vi "Semi Auto Intake Mode.vi"(9 "Current Intake Angle":dbl) -> (1 "Intake Open":bool, 2 "Intake Right Power":dbl, 3 "Intake Left Power":dbl, 4 "Intake Angle":dbl, 5 "Intake States":T1)   [LabVIEW 2017]
uses:
  Common Code/Intake States.ctl
  Robot Global Data.vi
  <vilib>/addons/control/pid/pid.llb/PID (DBL).vi
  <vilib>/addons/control/pid/NI_PID_pid.lvlib
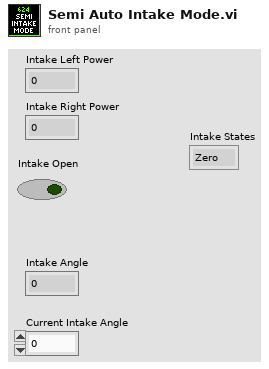
[diagram p1: front panel]
types:
  T1 = typedef "Intake States.ctl" = enum16{"Zero", "Override Angle", "Idle", "Drop Mid", "Drop Low", "Outtake", "Intake"}
  T2 = typedef "Drivetrain Settings Cluster.ctl" = cluster{"Gyro Steer PID Gains":T3, "Distance Drive PID Gains":T3, "Drive Tolerance":dbl, "Gyro Tolerance":dbl, "Gyro Output":dbl, "Distance Output":dbl, "Y Power Multiplier":dbl, "Turn Power Multiplier":dbl, "Creep Rate":dbl, "Constant Power":bool, "DT Mode Modifier":enum16{"None, Default", "Cube", "Square"}, "Left Encoder Tick Constant":dbl, "Right Encoder Tick Constant":dbl, "Shift Speed":dbl}
  T3 = typedef "PID Gains Cluster.ctl" = cluster{"Integral Time":dbl, "Proportional Gain":dbl, "Derivative Time":dbl}
  T4 = typedef "Intake Presets.ctl" = cluster{"Idle Angle":dbl, "Mid Angle":dbl, "Low Angle":dbl, "Outtake Power":dbl, "Intake Power":dbl, "Unstuck":dbl, "Angle Tolerance":dbl, "Max Angle":dbl, "Max Current":dbl, "Current Trip Time":dbl, "Reset Encoder?":bool, "Encoder Scale":dbl, "PID gains":cluster{"proportional gain (Kc)":dbl, "integral time (Ti, min)":dbl, "derivative time (Td, min)":dbl}, "output range":cluster{"output high":dbl, "output low":dbl}}
  T5 = typedef "Elevator Settings Cluster.ctl" = cluster{"Ground Height":dbl, "Switch Height":dbl, "Scale High Height ":dbl, "Scale Low Height":dbl, "Elevator PID Gains":T6, "Elevator Tolerance":dbl, "Reset Encoders":bool, "Encoder Scale":dbl, "Max Height":dbl, "Mid Height":dbl, "output range":cluster{"output high":dbl, "output low":dbl}}
  T6 = typedef "PID Gains.ctl" = cluster{"proportional gain (Kc)":dbl, "integral time (Ti, min)":dbl, "derivative time (Td, min)":dbl}
  T7 = cluster{"Drivetrain Settings Cluster":T2, "Intake Presets":T4, "Elevator Settings Cluster":T5}
  T8 = typedef "Elevator Status Cluster.ctl" = cluster{"Finished":bool, "Output":dbl, "Elevator State":T9, "Elevator Mode":T10, "Encoder Height":dbl, "Elevator Height":dbl, "At Bottom?":bool, "At Top?":bool}
  T9 = typedef "Elevator State.ctl" = enum16{"Idle", "Ground", "Mid", "Scale", "Switch"}
  T10 = typedef "Elevator Mode.ctl" = enum16{"Semi Auto", "Manual", "Auto"}
  T11 = typedef "Intake Command Cluster.ctl" = cluster{"Intake Mode":T12, "Intake States":T1, "Manual Roller Power":dbl, "Manual Close?":bool, "Manual Lift Power":dbl, "Override Lift?":bool, "Override Angle":dbl}
  T12 = typedef "Intake Mode.ctl" = enum16{"Auto", "Semi Auto", "Manual"}
  T13 = cluster{"proportional gain (Kc)":dbl, "integral time (Ti, min)":dbl, "derivative time (Td, min)":dbl}
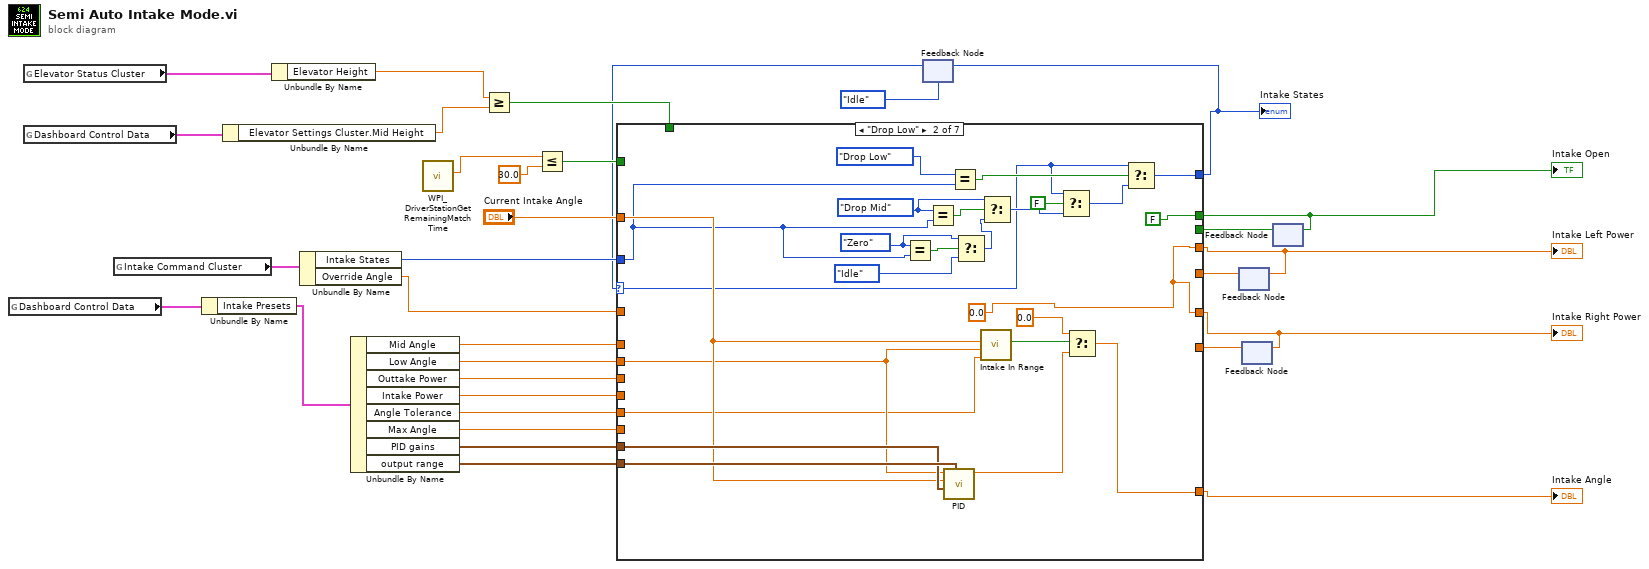
[diagram p0: block diagram]
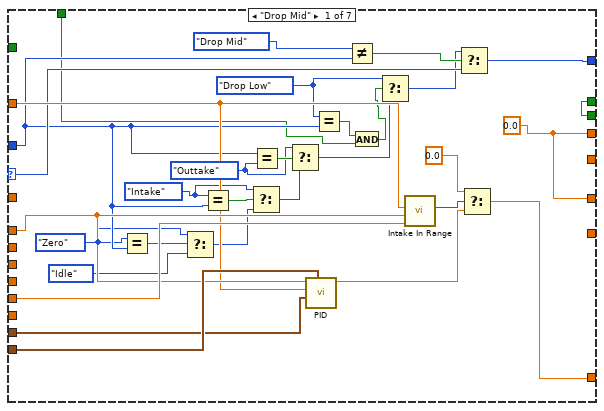
[diagram p2: hidden frame]
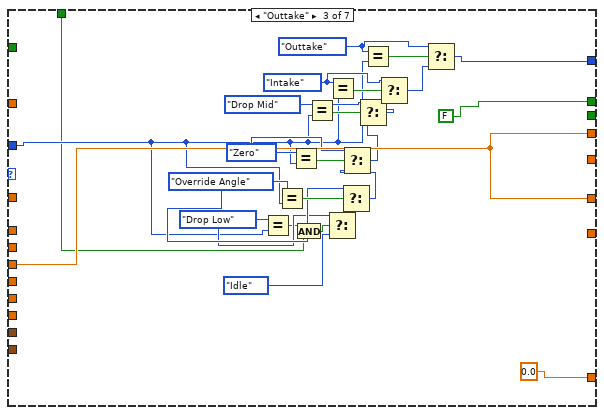
[diagram p3: hidden frame]
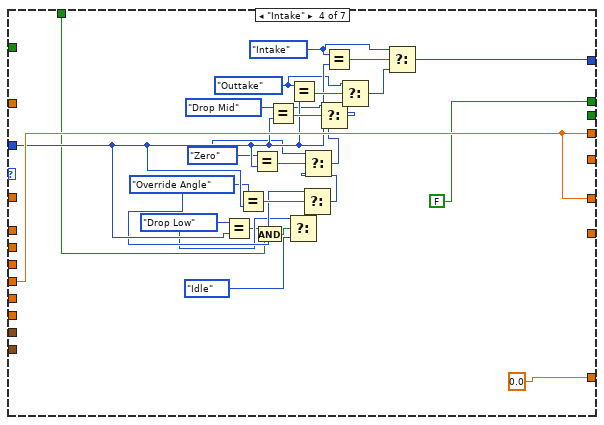
[diagram p4: hidden frame]
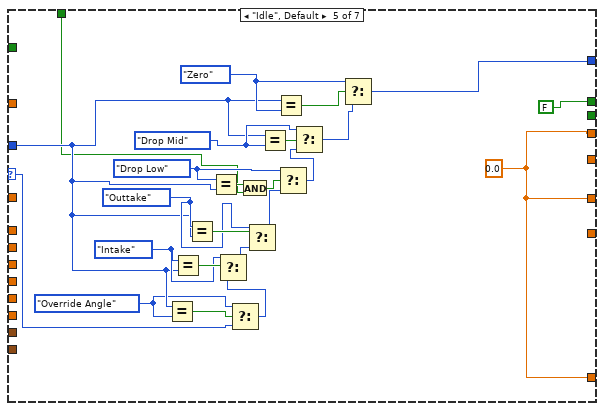
[diagram p5: hidden frame]
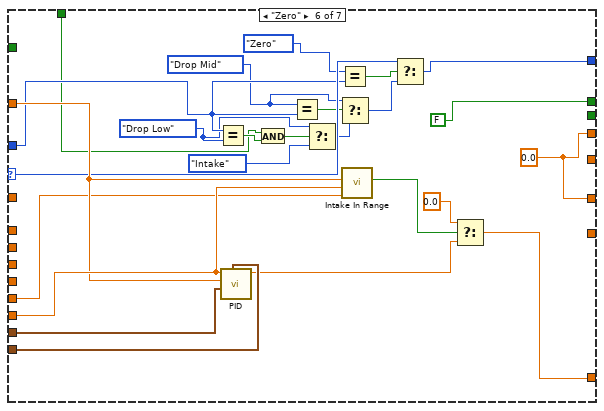
[diagram p6: hidden frame]
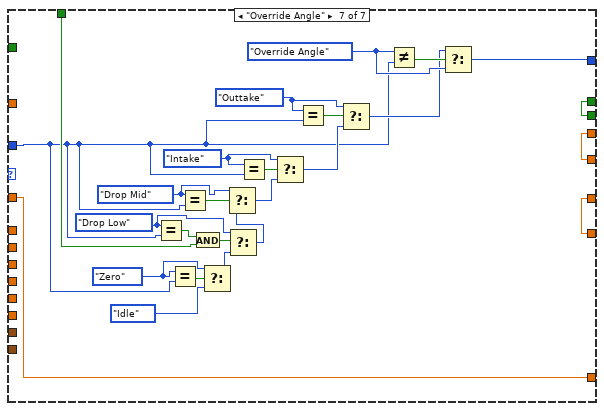
[diagram p7: hidden frame]
diagram:
  n1 = global read "Robot Global Data.vi" "Dashboard Control Data"() -> (w30:T7)
  n2 = global read "Robot Global Data.vi" "Elevator Status Cluster"() -> (w18:T8)
  n3 = global read "Robot Global Data.vi" "Dashboard Control Data"() -> (w17:T7)
  n4 = global read "Robot Global Data.vi" "Intake Command Cluster"() -> (w32:T11)
  n5 = Unbundle By Name(w30) -> ("Intake Presets"=w29:T4)
  n6 = Unbundle By Name(w17) -> ("Elevator Settings Cluster.Mid Height"=w15:dbl)
  n7 = Unbundle By Name(w18) -> ("Elevator Height"=w16:dbl)
  n8 = Unbundle By Name(w32) -> ("Intake States"=w31:T1, "Override Angle"=w7:dbl)
  n9 = Unbundle By Name(w29) -> ("Mid Angle"=w28:dbl, "Low Angle"=w27:dbl, "Outtake Power"=w26:dbl, "Intake Power"=w25:dbl, "Angle Tolerance"=w24:dbl, "Max Angle"=w23:dbl, "PID gains"=w22:T13, "output range"=w21:cluster{"output high":dbl, "output low":dbl})
  n10 = call <vilib>:"WPI_DriverStationGetRemainingMatchTime.vi"() -> ("Match Time(s)"=w13:sgl)  [unwired: 10 in, 1 out]
  n11 = Greater Or Equal?(x=w16, y=w15) -> (x >= y?=w14:bool)
  n12 = Less Or Equal?(x=w13, y=30.0) -> (x <= y?=w11:bool)
  n13 = feedback #1(Intake_States."Idle" ("Intake States")) -> (w8:T1)
  n14 = feedback #2() -> (w5:dbl)  [unwired: 1 in]
  n15 = feedback #3() -> (w3:dbl)  [unwired: 1 in]
  n16 = feedback #4() -> (w9:bool)  [unwired: 1 in]
  n17 = case shown="\"Drop Low\"" w8 {
    selector: w8 -> [w51 w73 _ _ w141 w175 _]
    tunnel: w31 -> [w41 w67 w91 w129 w147 w173 w193]
    tunnel: [w37 w71 w90 w114 w152 w164 w188] -> w1
    tunnel: [w33 FALSE FALSE FALSE FALSE FALSE w212] -> w10
    tunnel: [w54 w66 w112 w138 w148 w178 w211] -> w6
    tunnel: [w54 w66 w112 w138 w148 w178 w210] -> w4
    tunnel: [w55 w83 0.0 0.0 w148 w179 w213] -> w19
    tunnel: w28 -> [w60 _ _ _ _ _ _]
    tunnel: w27 -> [_ w81 _ _ _ _ _]
    tunnel: w26 -> [_ _ w112 _ _ _ _]
    tunnel: w25 -> [_ _ _ w138 _ _ _]
    tunnel: w24 -> [w61 w80 _ _ _ w183 _]
    tunnel: w23 -> [_ _ _ _ _ w185 _]
    tunnel: w22 -> [w62 w87 _ _ _ w187 _]
    tunnel: w21 -> [w63 w88 _ _ _ w186 _]
    tunnel: "Current Intake Angle" -> [w59 w82 _ _ _ w184 _]
    tunnel: w14 -> [w34 _ w89 w117 w145 w171 w198]
    tunnel: w11 -> [_ _ _ _ _ _ _]
    tunnel: w9 -> [w33 _ _ _ _ _ w212]
    tunnel: w7 -> [_ _ _ _ _ _ w213]
    tunnel: w5 -> [_ _ _ _ _ _ w211]
    tunnel: w3 -> [_ _ _ _ _ _ w210]
    frame "Drop Mid" {
      w40 = Intake_States."Zero" ("Intake States")
      w44 = Intake_States."Intake" ("Intake States")
      w48 = Intake_States."Outtake" ("Intake States")
      w50 = Intake_States."Drop Low" ("Intake States")
      w54 = 0.0
      n18 = Equal?(x=w40, y=w41) -> (x = y?=w42:bool)
      n19 = Select(t=w40, s=w42, f=Intake_States."Idle" ("Intake States")) -> (s? t:f=w38:T1)
      n20 = Equal?(x=w44, y=w41) -> (x = y?=w45:bool)
      n21 = Select(t=w44, s=w45, f=w38) -> (s? t:f=w43:T1)
      n22 = Equal?(x=w41, y=w48) -> (x = y?=w49:bool)
      n23 = Select(t=w48, s=w49, f=w43) -> (s? t:f=w47:T1)
      n24 = call-poly <vilib>:"PID.vi"("output range"=w63, "PID gains"=w62, "process variable"=w59, "setpoint"=w60) -> ("output"=w57:dbl)  [unwired: 6 in, 1 out]
      n25 = Equal?(x=w50, y=w41) -> (x = y?=w36:bool)
      n26 = Not Equal?(x=Intake_States."Drop Mid" ("Intake States"), y=w41) -> (x != y?=w52:bool)
      n27 = And(x=w36, y=w34) -> (x .and. y?=w35:bool)
      n28 = Select(t=w50, s=w35, f=w47) -> (s? t:f=w46:T1)
      n29 = call "Intake In Range.vi"("Angle Tolerance"=w61, "Target Height"=w60, "Actual Height"=w59) -> ("In Range?"=w58:bool)  [unwired: 8 in]
      n30 = Select(t=w46, s=w52, f=w51) -> (s? t:f=w37:T1)
      n31 = Select(t=0.0, s=w58, f=w57) -> (s? t:f=w55:dbl)
    }
    frame "Drop Low" {
      w66 = 0.0
      w70 = Intake_States."Zero" ("Intake States")
      w76 = Intake_States."Drop Mid" ("Intake States")
      n32 = Equal?(x=w70, y=w67) -> (x = y?=w75:bool)
      n33 = Equal?(x=w76, y=w67) -> (x = y?=w77:bool)
      n34 = call-poly <vilib>:"PID.vi"("output range"=w88, "PID gains"=w87, "process variable"=w82, "setpoint"=w81) -> ("output"=w85:dbl)  [unwired: 6 in, 1 out]
      n35 = Equal?(x=Intake_States."Drop Low" ("Intake States"), y=w67) -> (x = y?=w78:bool)
      n36 = Select(t=w70, s=w75, f=Intake_States."Idle" ("Intake States")) -> (s? t:f=w69:T1)
      n37 = call "Intake In Range.vi"("Angle Tolerance"=w80, "Target Height"=w81, "Actual Height"=w82) -> ("In Range?"=w86:bool)  [unwired: 8 in]
      n38 = Select(t=w76, s=w77, f=w69) -> (s? t:f=w74:T1)
      n39 = Select(t=w73, s=FALSE, f=w74) -> (s? t:f=w72:T1)
      n40 = Select(t=0.0, s=w86, f=w85) -> (s? t:f=w83:dbl)
      n41 = Select(t=w73, s=w78, f=w72) -> (s? t:f=w71:T1)
    }
    frame "Outtake" {
      w100 = Intake_States."Drop Low" ("Intake States")
      w101 = Intake_States."Override Angle" ("Intake States")
      w102 = Intake_States."Zero" ("Intake States")
      w103 = Intake_States."Drop Mid" ("Intake States")
      w104 = Intake_States."Intake" ("Intake States")
      w109 = Intake_States."Outtake" ("Intake States")
      n42 = Equal?(x=w100, y=w91) -> (x = y?=w94:bool)
      n43 = Equal?(x=w101, y=w91) -> (x = y?=w105:bool)
      n44 = Equal?(x=w102, y=w91) -> (x = y?=w106:bool)
      n45 = And(x=w94, y=w89) -> (x .and. y?=w93:bool)
      n46 = Equal?(x=w103, y=w91) -> (x = y?=w107:bool)
      n47 = Select(t=w100, s=w93, f=Intake_States."Idle" ("Intake States")) -> (s? t:f=w95:T1)
      n48 = Equal?(x=w104, y=w91) -> (x = y?=w108:bool)
      n49 = Select(t=w101, s=w105, f=w95) -> (s? t:f=w96:T1)
      n50 = Select(t=w102, s=w106, f=w96) -> (s? t:f=w97:T1)
      n51 = Select(t=w103, s=w107, f=w97) -> (s? t:f=w99:T1)
      n52 = Equal?(x=w109, y=w91) -> (x = y?=w110:bool)
      n53 = Select(t=w104, s=w108, f=w99) -> (s? t:f=w98:T1)
      n54 = Select(t=w109, s=w110, f=w98) -> (s? t:f=w90:T1)
    }
    frame "Intake" {
      w124 = Intake_States."Drop Low" ("Intake States")
      w125 = Intake_States."Override Angle" ("Intake States")
      w126 = Intake_States."Zero" ("Intake States")
      w127 = Intake_States."Drop Mid" ("Intake States")
      w128 = Intake_States."Outtake" ("Intake States")
      w134 = Intake_States."Intake" ("Intake States")
      n55 = Equal?(x=w124, y=w129) -> (x = y?=w118:bool)
      n56 = Equal?(x=w125, y=w129) -> (x = y?=w130:bool)
      n57 = Equal?(x=w126, y=w129) -> (x = y?=w131:bool)
      n58 = And(x=w118, y=w117) -> (x .and. y?=w116:bool)
      n59 = Equal?(x=w127, y=w129) -> (x = y?=w132:bool)
      n60 = Select(t=w124, s=w116, f=Intake_States."Idle" ("Intake States")) -> (s? t:f=w119:T1)
      n61 = Equal?(x=w128, y=w129) -> (x = y?=w133:bool)
      n62 = Select(t=w125, s=w130, f=w119) -> (s? t:f=w120:T1)
      n63 = Select(t=w126, s=w131, f=w120) -> (s? t:f=w121:T1)
      n64 = Select(t=w127, s=w132, f=w121) -> (s? t:f=w123:T1)
      n65 = Equal?(x=w134, y=w129) -> (x = y?=w135:bool)
      n66 = Select(t=w128, s=w133, f=w123) -> (s? t:f=w122:T1)
      n67 = Select(t=w134, s=w135, f=w122) -> (s? t:f=w114:T1)
    }
    frame "Idle", Default {
      w142 = Intake_States."Override Angle" ("Intake States")
      w148 = 0.0
      w155 = Intake_States."Intake" ("Intake States")
      w157 = Intake_States."Outtake" ("Intake States")
      w156 = Intake_States."Drop Low" ("Intake States")
      w149 = Intake_States."Drop Mid" ("Intake States")
      w161 = Intake_States."Zero" ("Intake States")
      n68 = Equal?(x=w147, y=w142) -> (x = y?=w143:bool)
      n69 = Equal?(x=w155, y=w147) -> (x = y?=w158:bool)
      n70 = Equal?(x=w157, y=w147) -> (x = y?=w159:bool)
      n71 = Equal?(x=w156, y=w147) -> (x = y?=w146:bool)
      n72 = Select(t=w142, s=w143, f=w141) -> (s? t:f=w140:T1)
      n73 = Select(t=w155, s=w158, f=w140) -> (s? t:f=w153:T1)
      n74 = And(x=w146, y=w145) -> (x .and. y?=w144:bool)
      n75 = Select(t=w157, s=w159, f=w153) -> (s? t:f=w154:T1)
      n76 = Equal?(x=w147, y=w149) -> (x = y?=w160:bool)
      n77 = Equal?(x=w147, y=w161) -> (x = y?=w162:bool)
      n78 = Select(t=w156, s=w144, f=w154) -> (s? t:f=w150:T1)
      n79 = Select(t=w149, s=w160, f=w150) -> (s? t:f=w151:T1)
      n80 = Select(t=w161, s=w162, f=w151) -> (s? t:f=w152:T1)
    }
    frame "Zero" {
      w169 = Intake_States."Drop Low" ("Intake States")
      w168 = Intake_States."Drop Mid" ("Intake States")
      w178 = 0.0
      n81 = Equal?(x=w173, y=w169) -> (x = y?=w172:bool)
      n82 = call-poly <vilib>:"PID.vi"("output range"=w186, "PID gains"=w187, "process variable"=w184, "setpoint"=w185) -> ("output"=w181:dbl)  [unwired: 6 in, 1 out]
      n83 = And(x=w171, y=w172) -> (x .and. y?=w170:bool)
      n84 = Equal?(x=w168, y=w173) -> (x = y?=w174:bool)
      n85 = Select(t=w169, s=w170, f=Intake_States."Intake" ("Intake States")) -> (s? t:f=w166:T1)
      n86 = Equal?(x=Intake_States."Zero" ("Intake States"), y=w173) -> (x = y?=w176:bool)
      n87 = Select(t=w168, s=w174, f=w166) -> (s? t:f=w167:T1)
      n88 = call "Intake In Range.vi"("Angle Tolerance"=w183, "Target Height"=w185, "Actual Height"=w184) -> ("In Range?"=w182:bool)  [unwired: 8 in]
      n89 = Select(t=w175, s=w176, f=w167) -> (s? t:f=w164:T1)
      n90 = Select(t=0.0, s=w182, f=w181) -> (s? t:f=w179:dbl)
    }
    frame "Override Angle" {
      w191 = Intake_States."Zero" ("Intake States")
      w196 = Intake_States."Drop Low" ("Intake States")
      w200 = Intake_States."Drop Mid" ("Intake States")
      w203 = Intake_States."Intake" ("Intake States")
      w207 = Intake_States."Outtake" ("Intake States")
      w206 = Intake_States."Override Angle" ("Intake States")
      n91 = Equal?(x=w196, y=w193) -> (x = y?=w199:bool)
      n92 = Equal?(x=w191, y=w193) -> (x = y?=w192:bool)
      n93 = Equal?(x=w200, y=w193) -> (x = y?=w201:bool)
      n94 = And(x=w199, y=w198) -> (x .and. y?=w197:bool)
      n95 = Select(t=w191, s=w192, f=Intake_States."Idle" ("Intake States")) -> (s? t:f=w190:T1)
      n96 = Select(t=w196, s=w197, f=w190) -> (s? t:f=w194:T1)
      n97 = Select(t=w200, s=w201, f=w194) -> (s? t:f=w195:T1)
      n98 = Equal?(x=w203, y=w193) -> (x = y?=w204:bool)
      n99 = Select(t=w203, s=w204, f=w195) -> (s? t:f=w202:T1)
      n100 = Equal?(x=w207, y=w193) -> (x = y?=w208:bool)
      n101 = Select(t=w207, s=w208, f=w202) -> (s? t:f=w205:T1)
      n102 = Not Equal?(x=w206, y=w193) -> (x != y?=w209:bool)
      n103 = Select(t=w205, s=w209, f=w206) -> (s? t:f=w188:T1)
    }
  }
  "Intake Left Power" <- w6
  "Intake Right Power" <- w4
  "Intake Open" <- w10
  "Intake Angle" <- w19
  "Intake States" <- w1
  n104 = feedback-in #1(w1) -> ()
  n105 = feedback-in #2(w6) -> ()
  n106 = feedback-in #3(w4) -> ()
  n107 = feedback-in #4(w10) -> ()
